vi "Main.vi"(9 "MICROS":T1, 10 "VISA resource name":refnum<visa-resource-name>, 11 "Module Admin":refnum<class "Delacor_lib_QMH_Cloneable Module Admin.lvclass">) -> ()   [LabVIEW 2019, in "MAIN.lvlib"]
doc: "This template is based off of the Queued Message Handler design pattern and the Queued Message Handler project template that ships with LabVIEW.\n\nThe main difference is that the queue is private to this module and communication between modules is performed via Broadcast and Request events.\n\nRequest events are wrapped in public API methods and are handled in the Event Handling Loop (EHL) of this VI. Any module can register for Broadcast events sent by this module. The EHL generates messages based on user interface actions.\n\nThe Message Handling Loop (MHL) processes messages generated by the EHL, or by other messages. The messages are string values, so new messages can be added easily to the Message Cases case structure in the MHL. Each message cluster can also provide an optional value for Message Data, which is a variant that can be converted to whatever message-specific data is required.\n_____\nBased on Delacor QMH Project Template 5.0.0.82."
uses:
  MAIN.lvlib
  <vilib>/Delacor/Delacor QMH/Libraries/Cloneable Module Admin_class/Delacor_lib_QMH_Cloneable Module Admin.lvclass
  C:/Program Files (x86)/National Instruments/LabVIEW 2019/vi.lib/Delacor/Delacor QMH/Libraries/Module Admin_class/Delacor_lib_QMH_Module Admin.lvclass
  MICROS.ctl
  Module Data--cluster.ctl
  ARDUINO/ARDUINO.lvclass
  D:/Repositorios Git/FINAL_AHORA_SI/SERIAL DEVICE/SERIAL DEVICE.lvclass
  <vilib>/Delacor/Delacor QMH/Libraries/Message Queue_class/Delacor_lib_QMH_Message Queue.lvclass/Delacor_lib_QMH_Message Queue.ctl
  <vilib>/Delacor/Delacor QMH/Libraries/Cloneable Module Admin_class/Delacor_lib_QMH_Cloneable Module Admin.lvclass/Delacor_lib_QMH_Cloneable Module Admin.ctl
  Stop Argument--cluster.ctl
  <vilib>/Delacor/Delacor QMH/Libraries/Module Admin_class/Delacor_lib_QMH_Module Admin.lvclass/Delacor_lib_QMH_Module Admin.ctl
  READ_ADC Argument--cluster.ctl
  READ_ADC (Reply Payload)--cluster.ctl
  READ PIN Argument--cluster.ctl
  READ PIN (Reply Payload)--cluster.ctl
  <vilib>/Utility/miscctls.llb/LVPointTypeDef.ctl
  SERIAL DEVICE/SERIAL DEVICE.lvclass/SERIAL DEVICE.ctl
  <vilib>/Delacor/Delacor QMH/Libraries/Message Queue_class/Delacor_lib_QMH_Enqueue Message (Single).vi
  <vilib>/Delacor/Delacor QMH/Libraries/Cloneable Module Admin_class/Delacor_lib_QMH_Get Module ID.vi
  <vilib>/Delacor/Delacor QMH/Libraries/Module Admin_class/Delacor_lib_QMH_Get External Launch.vi
  <vilib>/Utility/error.llb/Error Cluster From Error Code.vi
  <vilib>/ErrorRing/Error Ring.xnode
  <vilib>/Delacor/Delacor QMH/Libraries/Message Queue_class/Delacor_lib_QMH_Message Queue.lvclass
  SERIAL DEVICE/SERIAL DEVICE.lvclass
panel:
  out "Lectua PIN":string
  in  "Leer estado Pin":bool
  in  "Número de pin":u8
  in  "LEER ADC":bool
  out "LECTURA ADC":string
  in  "CANAL":u8
  in  "Simulate MHL Error":bool
  in  "Simulate EHL Error":bool
  out "error out":errorcluster
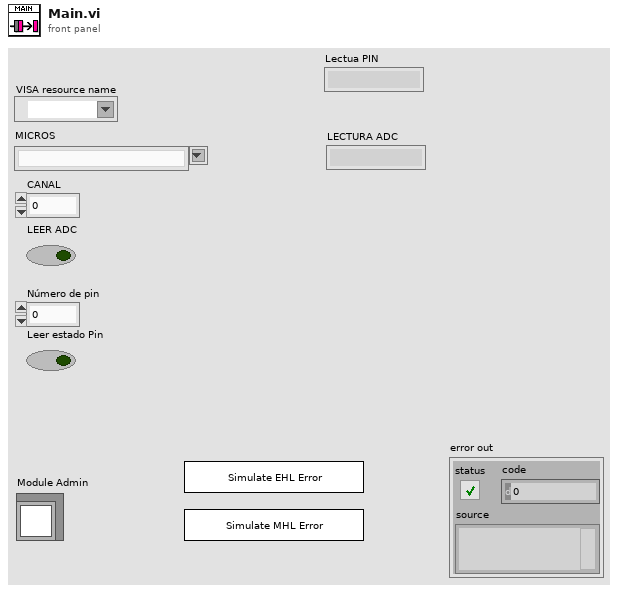
[diagram p1: front panel]
types:
  T1 = typedef "MICROS.ctl" = string
  T2 = typedef "MAIN.lvlib/Request Events--cluster.ctl" = cluster{"Stop Module":refnum<user-event>, "Show Panel":refnum<user-event>, "Hide Panel":refnum<user-event>, "Show Diagram":refnum<user-event>, "Get Module Execution Status":refnum<user-event>, "READ_ADC":refnum<user-event>, "READ PIN":refnum<user-event>}
  T3 = typedef "MAIN.lvlib/Module Data--cluster.ctl" = cluster{"Status":string, "SERIAL DEVICE":refnum<class "ARDUINO.lvclass">}
  T4 = enum32{"invalid lock state", "Not Locked", "Locked (No Password)", "Password-protected"}
  T5 = typedef "MAIN.lvlib/Stop Argument--cluster.ctl" = cluster{"Module ID":i32, "Origin":string, "Exit via Stop Module Req?":bool, "Wait for Module to stop?":bool}
  T6 = typedef "MAIN.lvlib/READ_ADC Argument--cluster.ctl" = cluster{"Module ID":i32, "CANAL":u8, "Wait Notifier":refnum<notifier>, "wait for reply":bool}
  T7 = typedef "MAIN.lvlib/READ PIN Argument--cluster.ctl" = cluster{"Module ID":i32, "CANAL PIN":u8, "Wait Notifier":refnum<notifier>, "wait for reply":bool}
  T8 = typedef "LVPointTypeDef.ctl" = cluster{"Horizontal":i16, "Vertical":i16}
  T9 = enum32{"Invalid", "Standard", "Closed", "Hidden", "Minimized", "Maximized"}
  T10 = typedef "MAIN.lvlib/READ_ADC (Reply Payload)--cluster.ctl" = cluster{"read buffer":string, "READ_ADC_error":errorcluster}
  T11 = typedef "MAIN.lvlib/READ PIN (Reply Payload)--cluster.ctl" = cluster{"READ BUFFER":string, "READ PIN_error":errorcluster}
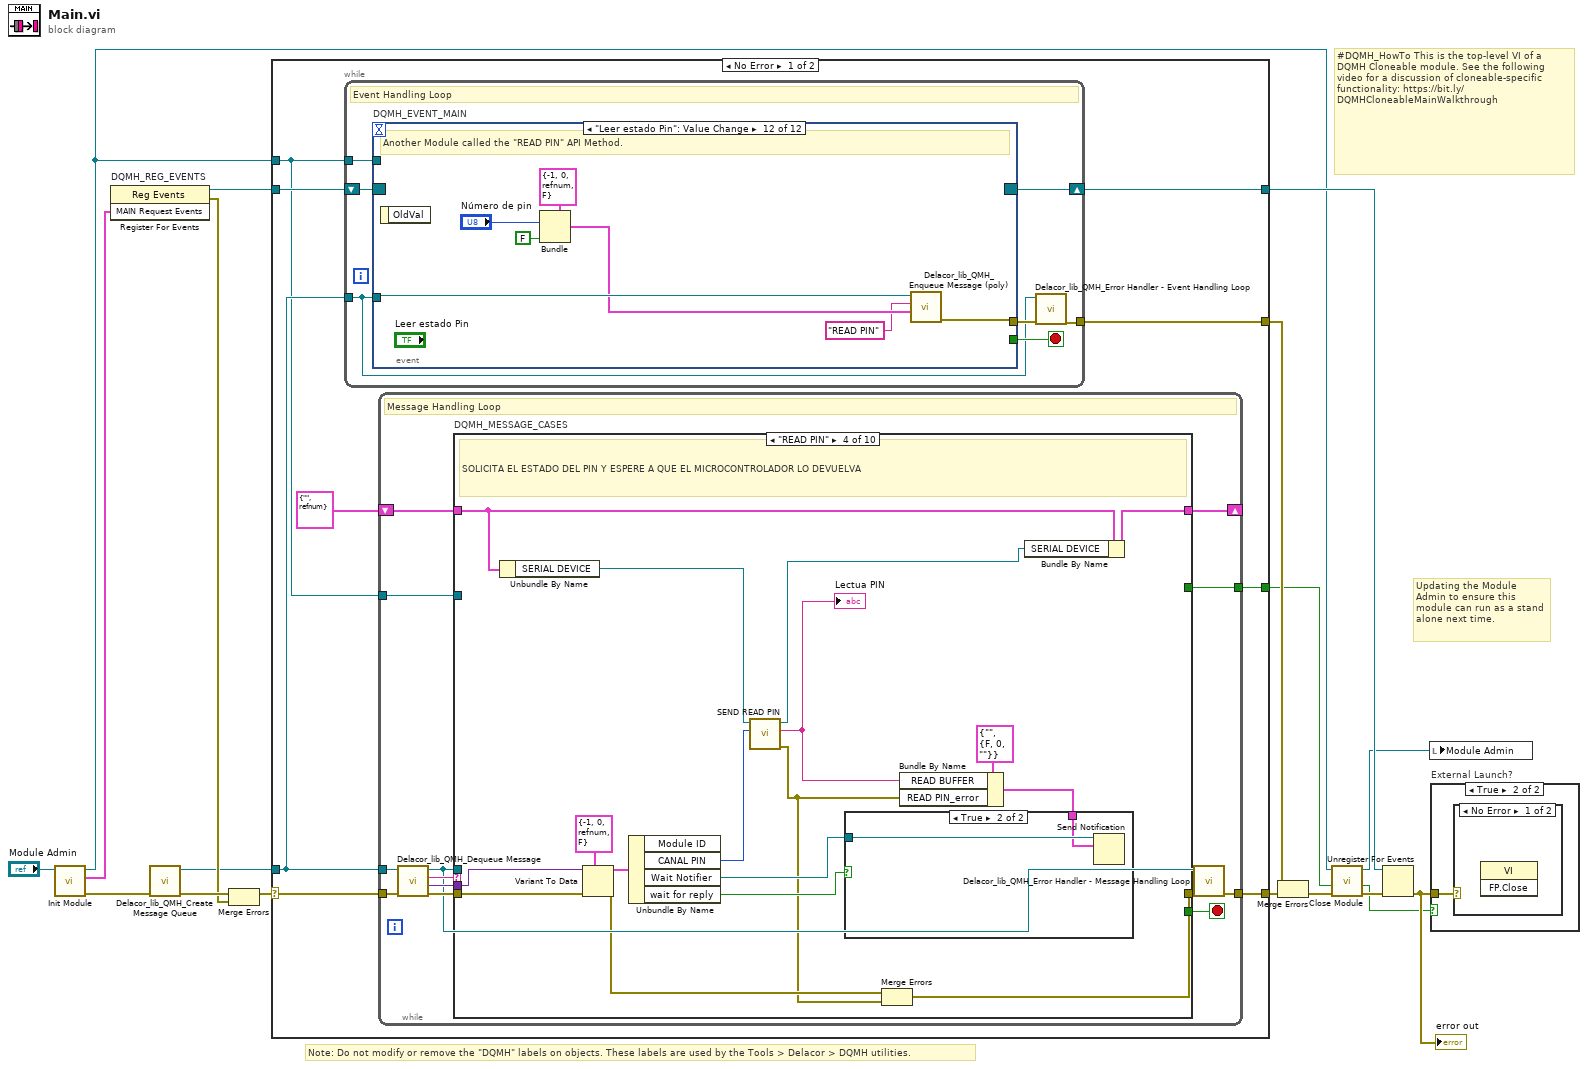
[diagram p0: block diagram]
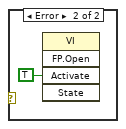
[diagram p3: hidden frame]
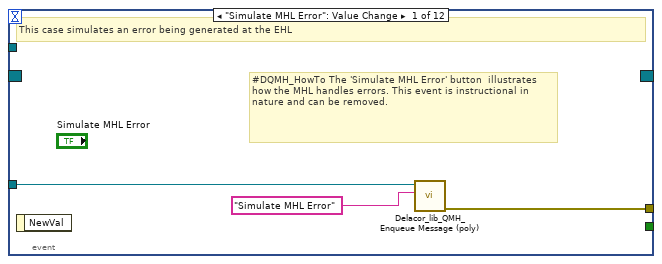
[diagram p4: hidden frame]
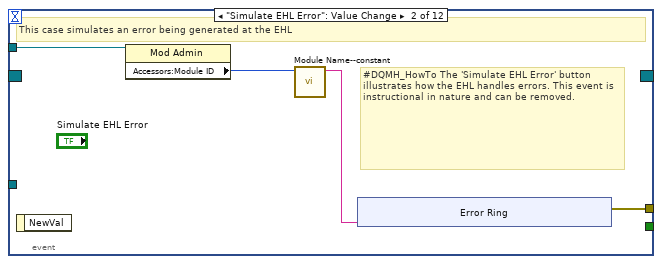
[diagram p5: hidden frame]
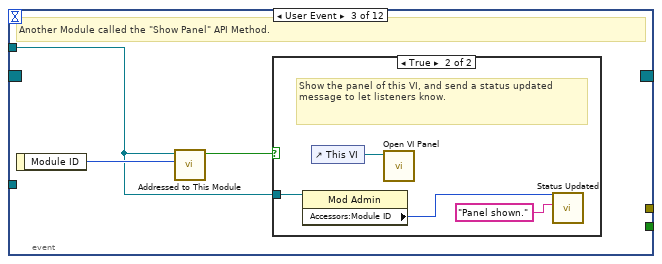
[diagram p6: hidden frame]
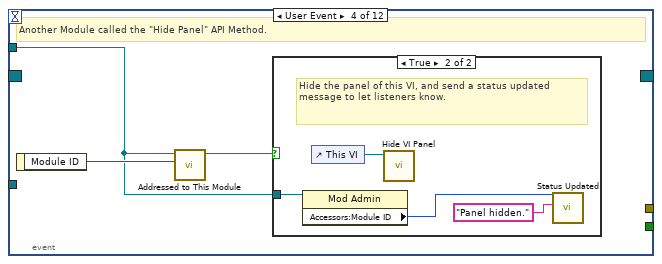
[diagram p8: hidden frame]
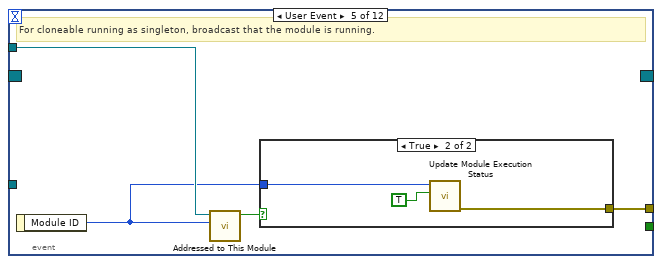
[diagram p10: hidden frame]
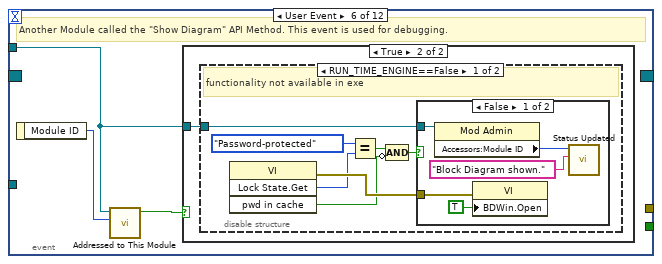
[diagram p12: hidden frame]
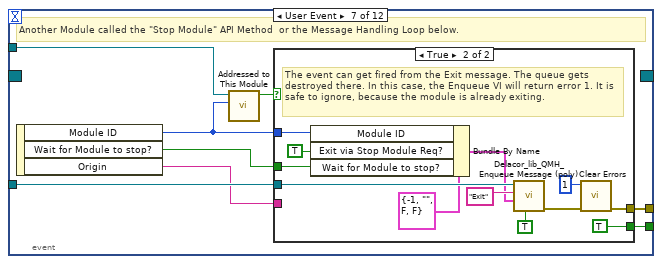
[diagram p16: hidden frame]
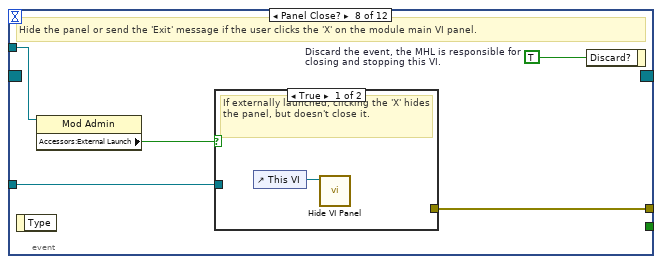
[diagram p18: hidden frame]
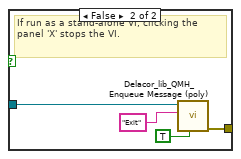
[diagram p19: hidden frame]
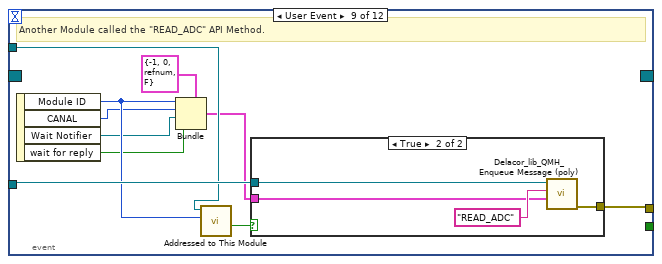
[diagram p20: hidden frame]
diagram:
  # "#DQMH_HowTo This is the top-level VI of a DQMH Cloneable module. See the following video for a discussion of cloneable-specific functionality: https://bit.ly/DQMHCloneableMainWalkthrough"
  # "Note: Do not modify or remove the \"DQMH\" labels on objects. These labels are used by the Tools > Delacor > DQMH utilities."
  # "Updating the Module Admin to ensure this module can run as a stand alone next time."
  n1 = call "Init Module.vi"("Cloneable Module Admin in"="Module Admin") -> ("error out"=w15:errorcluster, "MAIN Request Events"=w7:T2, "Cloneable Module Admin out"=w4:refnum<class "Delacor_lib_QMH_Cloneable Module Admin.lvclass">)  [unwired: 8 in]
  n2 = register-events "DQMH_REG_EVENTS"(w7) -> (reference out=w8:refnum<event-registration>, error out=w10:errorcluster)  [unwired: 2 in]
  n3 = call <vilib>:"Delacor_lib_QMH_Create Message Queue.vi"("error in (no error)"=w15) -> ("error out"=w12:errorcluster, "Message Queue"=w6:refnum<class "Delacor_lib_QMH_Message Queue.lvclass">)  [unwired: 9 in]
  n4 = Merge Errors(w12, w10) -> (w11:errorcluster)
  n5 = case shown="No Error" w11 {
    selector: w11 -> [w25 w313]
    tunnel: [w27 w312] -> w16
    tunnel: [w24 w320] -> w9
    tunnel: w8 -> [w22 w320]
    tunnel: w6 -> [w21 w311]
    tunnel: [w26 _] -> w17
    tunnel: w4 -> [w20 w316]
    tunnel: [w19 _] -> w2
    frame No Error {
      n6 = while {
        tunnel: w21 -> [w28]
        shift-right: [w31] -> w24
        shift-left: w22 -> [w32]
        tunnel: [w33] -> w26
        tunnel: w20 -> [w29]
        stop <- w30 stop-if-true
        # "Event Handling Loop"
        n7 = event "DQMH_EVENT_MAIN" shown="[11] \"Leer estado Pin\": Value Change" {
          selector: w32 -> [_ _ _ _ _ _ _ _ _ _ _ _]
          dyn-events: [_ _ _ _ _ _ _ _ _ _ _ _] -> w31
          timeout: _ -> [_ _ _ _ _ _ _ _ _ _ _ _]
          tunnel: [_ _ _ _ _ _ w89 _ _ _ _ _] -> w30
          tunnel: w28 -> [w36 _ _ _ _ _ w92 w107 w125 w136 w146 w157]
          tunnel: [w37 w41 _ _ w66 _ w93 w110 w116 w133 w137 w154] -> w34
          tunnel: w29 -> [_ w40 w49 w56 w64 w70 w91 w108 w123 _ w144 _]
          event "Simulate MHL Error": Value Change {
            # "#DQMH_HowTo The 'Simulate MHL Error' button  illustrates how the MHL handles errors. This event is instructional in nature and can be removed."
            # "This case simulates an error being generated at the EHL"
            n8 = event-data() -> ()  [unwired: 1 in, 1 out]
            n9 = call-poly <vilib>:"Delacor_lib_QMH_Enqueue Message (poly).vi"("Message"="Simulate MHL Error", "Message Queue in"=w36) -> ("error out"=w37:errorcluster)  [unwired: 8 in, 1 out]
          }
          event "Simulate EHL Error": Value Change {
            # "#DQMH_HowTo The 'Simulate EHL Error' button  illustrates how the EHL handles errors. This event is instructional in nature and can be removed."
            # "This case simulates an error being generated at the EHL"
            n10 = event-data() -> ()  [unwired: 1 in, 1 out]
            n11 = property class="Mod Admin"(reference=w40) -> ("Accessors:Module ID"=w39:i32)  [unwired: 1 in, 2 out]
            n12 = call "Module Name--constant.vi"("Module ID"=w39) -> ("Module Name"=w38:string)  [unwired: 10 in]
            n13 = xnode "Error Ring"("parameter 0"=w38) -> ("error out"=w41:errorcluster)
          }
          event User Event {
            # "Another Module called the \"Show Panel\" API Method."
            n14 = event-data() -> ("Module ID"=w50:i32)  [unwired: 1 in]
            n15 = call "Addressed to This Module.vi"("Module ID from Argument"=w50, "Module Admin"=w49) -> ("Addressed to this instance?"=w51:bool)  [unwired: 8 in, 1 out]
            n16 = case shown="True" w51 {
              tunnel: w49 -> [_ w53]
              frame False {
              }
              frame True {
                # "Show the panel of this VI, and send a status updated message to let listeners know."
                n17 = property class="Mod Admin"(reference=w53) -> ("Accessors:Module ID"=w52:i32)  [unwired: 1 in, 2 out]
                n18 = control-ref of="This VI"() -> (w55:refnum<vi>)
                n19 = call "Open VI Panel.vi"("VI"=w55) -> ()  [unwired: 10 in, 1 out]
                n20 = call "Status Updated.vi"("Status"="Panel shown." ("format string"), "Module ID"=w52) -> ()  [unwired: 9 in, 1 out]
              }
            }
          }
          event User Event {
            # "Another Module called the \"Hide Panel\" API Method."
            n21 = event-data() -> ("Module ID"=w57:i32)  [unwired: 1 in]
            n22 = call "Addressed to This Module.vi"("Module ID from Argument"=w57, "Module Admin"=w56) -> ("Addressed to this instance?"=w58:bool)  [unwired: 8 in, 1 out]
            n23 = case shown="True" w58 {
              tunnel: w56 -> [_ w60]
              frame False {
              }
              frame True {
                # "Hide the panel of this VI, and send a status updated message to let listeners know."
                n24 = property class="Mod Admin"(reference=w60) -> ("Accessors:Module ID"=w59:i32)  [unwired: 1 in, 2 out]
                n25 = control-ref of="This VI"() -> (w62:refnum<vi>)
                n26 = call "Hide VI Panel.vi"("VI"=w62) -> ()  [unwired: 10 in, 1 out]
                n27 = call "Status Updated.vi"("Status"="Panel hidden." ("format string"), "Module ID"=w59) -> ()  [unwired: 9 in, 1 out]
              }
            }
          }
          event User Event {
            # "For cloneable running as singleton, broadcast that the module is running."
            n28 = event-data() -> ("Module ID"=w63:i32)  [unwired: 1 in]
            n29 = call "Addressed to This Module.vi"("Module ID from Argument"=w63, "Module Admin"=w64) -> ("Addressed to this instance?"=w65:bool)  [unwired: 8 in, 1 out]
            n30 = case shown="True" w65 {
              tunnel: [_ w69] -> w66
              tunnel: w63 -> [_ w68]
              frame False {
              }
              frame True {
                n31 = call "Update Module Execution Status.vi"("Running?"=TRUE, "Module ID"=w68) -> ("error out"=w69:errorcluster)  [unwired: 9 in]
              }
            }
          }
          event User Event {
            # "Another Module called the \"Show Diagram\" API Method. This event is used for debugging."
            n32 = event-data() -> ("Module ID"=w71:i32)  [unwired: 1 in]
            n33 = call "Addressed to This Module.vi"("Module ID from Argument"=w71, "Module Admin"=w70) -> ("Addressed to this instance?"=w72:bool)  [unwired: 8 in, 1 out]
            n34 = case shown="True" w72 {
              tunnel: w70 -> [_ w73]
              frame False {
              }
              frame True {
                n35 = disable-structure shown="RUN_TIME_ENGINE==False" {
                  disable-tunnel: w73 -> [w74 _]
                  frame condition #0 (active) {
                    # "functionality not available in exe"
                    n36 = invoke class="VI" method="Lock State.Get"() -> (error out=w80:errorcluster, "Get Lock State"=w79:T4, "pwd in cache"=w76:bool)  [unwired: 4 in, 1 out]
                    n37 = Equal?(x=T4."Password-protected", y=w79) -> (x = y?=w77:bool)
                    n38 = Compound Arithmetic op=AND(w77, invert w76) -> (w75:bool)
                    n39 = case shown="False" w75 {
                      tunnel: w80 -> [w85 _]
                      tunnel: w74 -> [w82 _]
                      frame False {
                        n40 = property class="Mod Admin"(reference=w82) -> ("Accessors:Module ID"=w81:i32)  [unwired: 1 in, 2 out]
                        n41 = property class="VI"(error in=w85, "BDWin.Open"=TRUE ("Block Diagram Window:Open")) -> ()  [unwired: 1 in, 2 out]
                        n42 = call "Status Updated.vi"("Status"="Block Diagram shown." ("format string"), "Module ID"=w81) -> ()  [unwired: 9 in, 1 out]
                      }
                      frame True {
                        # "Password-protected VI, and the password is not in the cache. Do not show the diagram."
                      }
                    }
                  }
                  frame condition #1 {
                  }
                }
              }
            }
          }
          event User Event {
            # "Another Module called the \"Stop Module\" API Method  or the Message Handling Loop below."
            n43 = event-data() -> ("Module ID"=w87:i32, "Wait for Module to stop?"=w88:bool, "Origin"=w86:string)  [unwired: 1 in]
            n44 = call "Addressed to This Module.vi"("Module ID from Argument"=w87, "Module Admin"=w91) -> ("Addressed to this instance?"=w90:bool)  [unwired: 8 in, 1 out]
            n45 = case shown="True" w90 {
              tunnel: [_ w104] -> w93
              tunnel: w92 -> [_ w100]
              tunnel: [_ TRUE] -> w89
              tunnel: w88 -> [_ w95]
              tunnel: w87 -> [_ w97]
              tunnel: w86 -> [_ _]
              frame False {
              }
              frame True {
                # "The event can get fired from the Exit message. The queue gets destroyed there. In this case, the Enqueue VI will return error 1. It is safe to ignore, because the module is already exiting."
                n46 = Bundle By Name(cluster=T5 {"Module ID"=-1, "Origin"="", "Exit via Stop Module Req?"=FALSE, "Wait for Module to stop?"=FALSE} ("Stop Argument"), "Module ID"=w97, "Exit via Stop Module Req?"=TRUE, "Wait for Module to stop?"=w95) -> (w94:T5)
                n47 = call-poly <vilib>:"Delacor_lib_QMH_Enqueue Message (poly).vi"("Priority Message? (F)"=TRUE, "Message Data"=w94, "Message"="Exit", "Message Queue in"=w100) -> ("error out"=w105:errorcluster)  [unwired: 6 in, 1 out]
                n48 = call <vilib>:"Clear Errors.vi"("error in (no error)"=w105, "specific error code to clear (0: all)"=1) -> ("error out"=w104:errorcluster)  [unwired: 4 in, 1 out]
              }
            }
          }
          event Panel Close? {
            w109 = TRUE  # Discard the event, the MHL is responsible for closing and stopping this VI.
            # "Hide the panel or send the 'Exit' message if the user clicks the 'X' on the module main VI panel."
            n49 = event-data() -> ()  [unwired: 1 in, 1 out]
            n50 = property class="Mod Admin"(reference=w108) -> ("Accessors:External Launch"=w106:bool)  [unwired: 1 in, 2 out]
            n51 = case shown="True" w106 {
              tunnel: w107 -> [_ w114]
              tunnel: [_ w115] -> w110
              frame True {
                # "If externally launched, clicking the 'X' hides the panel, but doesn't close it."
                n52 = control-ref of="This VI"() -> (w111:refnum<vi>)
                n53 = call "Hide VI Panel.vi"("VI"=w111) -> ()  [unwired: 10 in, 1 out]
              }
              frame False {
                # "If run as a stand-alone VI, clicking the panel 'X' stops the VI."
                n54 = call-poly <vilib>:"Delacor_lib_QMH_Enqueue Message (poly).vi"("Priority Message? (F)"=TRUE, "Message"="Exit", "Message Queue in"=w114) -> ("error out"=w115:errorcluster)  [unwired: 7 in, 1 out]
              }
            }
            n55 = event-data("Discard?"=w109) -> ()  [unwired: 1 in, 1 out]
          }
          event User Event {
            # "Another Module called the \"READ_ADC\" API Method."
            n56 = event-data() -> ("Module ID"=w120:i32, "CANAL"=w119:u8, "Wait Notifier"=w118:refnum<notifier>, "wait for reply"=w117:bool)  [unwired: 1 in]
            n57 = Bundle(cluster=T6 {"Module ID"=-1, "CANAL"=0, "Wait Notifier"=refnum, "wait for reply"=FALSE} ("READ_ADC Argument"), "Module ID"=w120, "CANAL"=w119, "Wait Notifier"=w118, "wait for reply"=w117) -> (w121:T6)
            n58 = call "Addressed to This Module.vi"("Module ID from Argument"=w120, "Module Admin"=w123) -> ("Addressed to this instance?"=w124:bool)  [unwired: 8 in, 1 out]
            n59 = case shown="True" w124 {
              tunnel: w125 -> [_ w129]
              tunnel: w121 -> [_ w127]
              tunnel: [_ w126] -> w116
              frame False {
              }
              frame True {
                n60 = call-poly <vilib>:"Delacor_lib_QMH_Enqueue Message (poly).vi"("Message Data"=w127, "Message"="READ_ADC", "Message Queue in"=w129) -> ("error out"=w126:errorcluster)  [unwired: 7 in, 1 out]
              }
            }
          }
          event "LEER ADC": Value Change {
            # "Another Module called the \"READ_ADC\" API Method."
            n61 = event-data() -> ()  [unwired: 1 in, 2 out]
            n62 = Bundle(cluster=T6 {"Module ID"=-1, "CANAL"=0, "Wait Notifier"=refnum, "wait for reply"=FALSE} ("READ_ADC Argument"), "CANAL"="CANAL", "wait for reply"=FALSE) -> (w134:T6)  [unwired: 2 in]
            n63 = call-poly <vilib>:"Delacor_lib_QMH_Enqueue Message (poly).vi"("Message Data"=w134, "Message"="READ_ADC", "Message Queue in"=w136) -> ("error out"=w133:errorcluster)  [unwired: 7 in, 1 out]
          }
          event User Event {
            # "Another Module called the \"READ PIN\" API Method."
            n64 = event-data() -> ("Module ID"=w141:i32, "CANAL PIN"=w140:u8, "Wait Notifier"=w139:refnum<notifier>, "wait for reply"=w138:bool)  [unwired: 1 in]
            n65 = Bundle(cluster=T7 {"Module ID"=-1, "CANAL PIN"=0, "Wait Notifier"=refnum, "wait for reply"=FALSE} ("READ PIN Argument"), "Module ID"=w141, "CANAL PIN"=w140, "Wait Notifier"=w139, "wait for reply"=w138) -> (w142:T7)
            n66 = call "Addressed to This Module.vi"("Module ID from Argument"=w141, "Module Admin"=w144) -> ("Addressed to this instance?"=w145:bool)  [unwired: 8 in, 1 out]
            n67 = case shown="True" w145 {
              tunnel: w146 -> [_ w150]
              tunnel: w142 -> [_ w148]
              tunnel: [_ w147] -> w137
              frame False {
              }
              frame True {
                n68 = call-poly <vilib>:"Delacor_lib_QMH_Enqueue Message (poly).vi"("Message Data"=w148, "Message"="READ PIN", "Message Queue in"=w150) -> ("error out"=w147:errorcluster)  [unwired: 7 in, 1 out]
              }
            }
          }
          event "Leer estado Pin": Value Change {
            # "Another Module called the \"READ PIN\" API Method."
            n69 = event-data() -> ()  [unwired: 1 in, 1 out]
            n70 = Bundle(cluster=T7 {"Module ID"=-1, "CANAL PIN"=0, "Wait Notifier"=refnum, "wait for reply"=FALSE} ("READ PIN Argument"), "CANAL PIN"="Número de pin", "wait for reply"=FALSE) -> (w155:T7)  [unwired: 2 in]
            n71 = call-poly <vilib>:"Delacor_lib_QMH_Enqueue Message (poly).vi"("Message Data"=w155, "Message"="READ PIN", "Message Queue in"=w157) -> ("error out"=w154:errorcluster)  [unwired: 7 in, 1 out]
          }
        }
        n72 = call-dynamic "Delacor_lib_QMH_Error Handler - Event Handling Loop.vi"("error in (no error)"=w34, "Message Queue in"=w28) -> ("dup error in"=w33:errorcluster)  [unwired: 8 in, 1 out]
      }
      n73 = while {
        tunnel: w21 -> [w161]
        shift-right: [w165] -> _
        shift-left: T3 {"Status"="", "SERIAL DEVICE"=refnum} ("Data Cluster") -> [w166]
        tunnel: w25 -> [w169]
        tunnel: [w167] -> w27
        tunnel: w20 -> [w159]
        tunnel: [w158] -> w19
        stop <- w164 stop-if-true
        # "Message Handling Loop"
        n74 = call-dynamic "Delacor_lib_QMH_Dequeue Message.vi"("error in (no error)"=w169, "Message Queue in"=w161) -> ("error out"=w168:errorcluster, "Message Data"=w162:variant, "Message"=w163:string, "Message Queue out"=w160:refnum<class "Delacor_lib_QMH_Message Queue.lvclass">)  [unwired: 6 in]
        n75 = case "DQMH_MESSAGE_CASES" shown="\"READ PIN\"" w163 {
          selector: w163 -> [_ _ _ _ _ _ _ _ _ w298]
          tunnel: w160 -> [_ _ _ _ _ _ w248 _ w288 _]
          tunnel: w168 -> [w195 w200 w219 w238 w243 w245 w257 w270 w294 w300]
          tunnel: [w193 w200 w210 w229 w242 w245 w253 w269 w291 w301] -> w170
          tunnel: w166 -> [w186 w199 w206 w227 w241 w244 w252 w267 w279 w299]
          tunnel: [w185 w199 w205 w228 w241 w244 w252 w267 w279 w299] -> w165
          tunnel: [_ _ _ _ _ _ _ _ w287 _] -> w164
          tunnel: w162 -> [_ _ w217 w236 _ _ w251 _ w285 _]
          tunnel: w159 -> [w180 _ _ _ _ _ w250 w265 w281 w296]
          tunnel: [_ _ _ _ _ _ _ _ w283 _] -> w158
          frame "Initialize" {
            # "Initialize - Any operation that needs to be done before the module can receive messages. Synchronize Caller Events.vi will inform Start Module.vi that the module has launched and is ready to receive messages. Module Did Init.vi will broadcast that the module initialized."
            n76 = call "Synchronize Caller Events.vi"("error in (no error)"=w195, "Module Admin"=w180) -> ("error out"=w194:errorcluster, "Module Admin out"=w179:refnum<class "Delacor_lib_QMH_Cloneable Module Admin.lvclass">)  [unwired: 8 in]
            n77 = property class="Mod Admin"(reference=w179) -> ("Accessors:Module ID"=w182:i32, "Accessors:External Launch"=w181:bool)  [unwired: 1 in, 2 out]
            n78 = case shown="\"A\"" "MICROS" {
              tunnel: [_ refnum<class "ARDUINO.lvclass"> refnum ("ARDUINO.lvclass")] -> w177
              frame "False", Default {
              }
              frame "A" {
              }
            }
            n79 = call "Module Name--constant.vi"("Module ID"=w182) -> ("Module Name"=w190:string)  [unwired: 10 in]
            n80 = call "Write MICROS.vi"("MICROS"="MICROS", "SERIAL DEVICE in"=w177) -> ("SERIAL DEVICE out"=w175:refnum<class "ARDUINO.lvclass">)  [unwired: 8 in, 1 out]
            n81 = property class="VI"("Front Panel.Title"=w190) -> (reference out=w192:refnum<vi>, error out=w197:errorcluster)  [unwired: 2 in]
            n82 = Select(t=T9."Hidden" ("State"), s=w181, f=T9."Standard" ("State")) -> (s? t:f=w187:T9)
            n83 = VISA Open(VISA resource name="VISA resource name") -> (VISA resource name=w171:refnum<visa-resource-name>)  [unwired: 4 in, 1 out]
            n84 = invoke class="VI" method="FP.Open"(reference=w192, error in=w197, "State"=w187) -> (reference out=w191:refnum<vi>, error out=w196:errorcluster)  [unwired: 2 in, 3 out]
            n85 = call "Module Name--constant.vi"("Module ID"=w182) -> ("Module Name"=w183:string)  [unwired: 10 in]
            n86 = call "Write VISA resource name.vi"("VISA resource name"=w171, "SERIAL DEVICE in"=w175) -> ("SERIAL DEVICE out"=w174:refnum<class "ARDUINO.lvclass">)  [unwired: 8 in, 1 out]
            n87 = call-dynamic "INIT.vi"("SERIAL DEVICE in"=w174) -> ("SERIAL DEVICE out"=w172:refnum<class "ARDUINO.lvclass">)  [unwired: 9 in, 1 out]
            n88 = invoke class="VI" method="FP.Center"(reference=w191, error in=w196) -> ()  [unwired: 1 in, 3 out]
            n89 = call "Module Did Init.vi"("error in (no error)"=w194, "Initialized?"=TRUE, "Origin"=w183, "Module ID"=w182) -> ("error out"=w193:errorcluster)  [unwired: 7 in]
            n90 = Bundle By Name(cluster=w186, "SERIAL DEVICE"=w172) -> (w185:T3)
            n91 = property on="Pane" class="Pane"("Origin"=T8 {"Horizontal"=0, "Vertical"=0}) -> ()  [unwired: 2 in, 2 out]
          }
          frame "--- Module Specific ---" {
            # "Separator -- The following cases handle messages specific to this Module."
          }
          frame "READ_ADC" {
            # "MANDA LEER EL ADC Y ESPERA A QUE EL MICRO RESPONDA LO ESPERADO"
            n92 = Unbundle By Name(w206) -> ("SERIAL DEVICE"=w207:refnum<class "ARDUINO.lvclass">)
            n93 = Variant To Data(error in=w219, type=T6 {"Module ID"=-1, "CANAL"=0, "Wait Notifier"=refnum, "wait for reply"=FALSE} ("READ_ADC Argument"), Variant=w217) -> (data=w215:T6, error out=w218:errorcluster)
            n94 = Unbundle By Name(w215) -> ("CANAL"=w209:u8, "Wait Notifier"=w214:refnum<notifier>, "wait for reply"=w213:bool)  [unwired: 1 out]
            n95 = call-dynamic "SEND ADC.vi"("CANAL"=w209, "SERIAL DEVICE in"=w207) -> ("error out"=w208:errorcluster, "read buffer"=w203:string, "SERIAL DEVICE out"=w204:refnum<class "ARDUINO.lvclass">)  [unwired: 7 in]
            n96 = Match Pattern(string=w203, regular expression=";") -> (before substring=→"LECTURA ADC":string)  [unwired: 1 in, 3 out]
            n97 = Bundle By Name(cluster=T10 {"read buffer"="", "READ_ADC_error"={"status"=FALSE, "code"=0, "source"=""}} ("READ_ADC (Reply Payload)"), "read buffer"=w203, "READ_ADC_error"=w208) -> (w212:T10)
            n98 = case shown="True" w213 {
              tunnel: w214 -> [_ w221]
              tunnel: w212 -> [_ w220]
              frame False {
              }
              frame True {
                n99 = Send Notification(notification=w220, notifier=w221) -> ()  [unwired: 1 in, 2 out]
              }
            }
            n100 = Merge Errors(w218, w208) -> (w210:errorcluster)
            n101 = Bundle By Name(cluster=w206, "SERIAL DEVICE"=w204) -> (w205:T3)
          }
          frame "READ PIN" {
            # "SOLICITA EL ESTADO DEL PIN Y ESPERE A QUE EL MICROCONTROLADOR LO DEVUELVA"
            n102 = Unbundle By Name(w227) -> ("SERIAL DEVICE"=w224:refnum<class "ARDUINO.lvclass">)
            n103 = Variant To Data(error in=w238, type=T7 {"Module ID"=-1, "CANAL PIN"=0, "Wait Notifier"=refnum, "wait for reply"=FALSE} ("READ PIN Argument"), Variant=w236) -> (data=w234:T7, error out=w237:errorcluster)
            n104 = Unbundle By Name(w234) -> ("CANAL PIN"=w223:u8, "Wait Notifier"=w233:refnum<notifier>, "wait for reply"=w232:bool)  [unwired: 1 out]
            n105 = call-dynamic "SEND READ PIN.vi"("CANAL"=w223, "SERIAL DEVICE in"=w224) -> ("error out"=w222:errorcluster, "read buffer"=w226:string, "SERIAL DEVICE out"=w225:refnum<class "ARDUINO.lvclass">)  [unwired: 7 in]
            "Lectua PIN" <- w226
            n106 = Merge Errors(w237, w222) -> (w229:errorcluster)
            n107 = Bundle By Name(cluster=T11 {"READ BUFFER"="", "READ PIN_error"={"status"=FALSE, "code"=0, "source"=""}} ("READ PIN (Reply Payload)"), "READ BUFFER"=w226, "READ PIN_error"=w222) -> (w231:T11)
            n108 = case shown="True" w232 {
              tunnel: w233 -> [_ w240]
              tunnel: w231 -> [_ w239]
              frame False {
              }
              frame True {
                n109 = Send Notification(notification=w239, notifier=w240) -> ()  [unwired: 1 in, 2 out]
              }
            }
            n110 = Bundle By Name(cluster=w227, "SERIAL DEVICE"=w225) -> (w228:T3)
          }
          frame "---Copy This Frame---" {
            # "Duplicate this frame when creating new messages.  Change this comment in the duplicated frame to describe this message."
            n111 = Merge Errors(w243) -> (w242:errorcluster)
          }
          frame "--- Exit and Error Handling---" {
            # "Separator - the following cases handle errors and exit messages."
          }
          frame "Error" {
            # "#CodeRecommended - If you ever change the name of this \"Error\" message, you'll need to update the name in the Check Loop Error.vi as well."
            # "#CodeRecommended - If the module is running in standalone mode (External Launch = FALSE), this code will pop up an error dialog and call the 'Exit' message if an error occurs. Add more fine-grained error handling here."
            # "Error - Check the error message data and respond accordingly. This message is sent by the \"Error Handler\" VIs at the end of each loop in this application."
            n112 = property class="Mod Admin"(reference=w250) -> ("Accessors:External Launch"=w249:bool, "Accessors:Module ID"=w246:i32)  [unwired: 1 in, 2 out]
            n113 = Variant To Data(error in=w257, type=errorcluster {"status"=FALSE, "code"=0, "source"=""} ("error constant"), Variant=w251) -> (data=w258:errorcluster, error out=w255:errorcluster)
            n114 = call "Module Name--constant.vi"("Module ID"=w246) -> ("Module Name"=w247:string)  [unwired: 10 in]
            n115 = call "Error Reported.vi"("Additional Information"=w247, "Error"=w258, "Module ID"=w246) -> ()  [unwired: 8 in, 1 out]
            n116 = case shown="False" w249 {
              tunnel: [w263 _] -> w254
              tunnel: w248 -> [w261 _]
              tunnel: w258 -> [w262 _]
              frame False {
                # "If the module is running standalone, then pop up an error dialog and call the \"Exit\" message."
                n117 = call <vilib>:"Simple Error Handler.vi"("error in (no error)"=w262) -> ()  [unwired: 4 in, 5 out]
                n118 = call-poly <vilib>:"Delacor_lib_QMH_Enqueue Message (poly).vi"("Priority Message? (F)"=TRUE, "Message"="Exit", "Message Queue in"=w261) -> ("error out"=w263:errorcluster)  [unwired: 7 in, 1 out]
              }
              frame True {
                # "If the module was launched externally, calling the Error Reported broadcast VI is the only action performed by the \"Error\" message. The module's caller can then process the error appropriately."
              }
            }
            n119 = Merge Errors(w255, w254) -> (w253:errorcluster)
            n120 = local write "error out"(w253) -> ()
          }
          frame "Simulate MHL Error" {
            # "#DQMH_HowTo The 'Simulate MHL Error' button  illustrates how the MHL handles errors. This event is instructional in nature and can be removed."
            # "Simulate an error occurring at the MHL"
            n121 = property class="Mod Admin"(reference=w265) -> ("Accessors:Module ID"=w266:i32)  [unwired: 1 in, 2 out]
            n122 = call "Module Name--constant.vi"("Module ID"=w266) -> ("Module Name"=w264:string)  [unwired: 10 in]
            n123 = xnode "Error Ring"("parameter 0"=w264) -> ("error out"=w268:errorcluster)
            n124 = Merge Errors(w270, w268) -> (w269:errorcluster)
          }
          frame "Exit" {
            w286 = 91  # 91: not all Exit messages will have an argument
            w287 = TRUE  # Stop the VI
            # "Release the message queue reference"
            # "Exit - Exit the application."
            n125 = Variant To Data(error in=w294, type=T5 {"Module ID"=-1, "Origin"="", "Exit via Stop Module Req?"=FALSE, "Wait for Module to stop?"=FALSE} ("Stop Argument"), Variant=w285) -> (data=w282:T5, error out=w289:errorcluster)
            n126 = Unbundle By Name(w279) -> ("SERIAL DEVICE"=w278:refnum<class "ARDUINO.lvclass">)
            n127 = call <vilib>:"Clear Errors.vi"("error in (no error)"=w289, "specific error code to clear (0: all)"=w286) -> ("error out"=w293:errorcluster)  [unwired: 4 in, 1 out]
            n128 = call-dynamic "CLOSE.vi"("SERIAL DEVICE in"=w278) -> ()  [unwired: 9 in, 2 out]
            n129 = control-ref of="This VI"() -> (w280:refnum<vi>)
            n130 = call-dynamic "Delacor_lib_QMH_Release Message Queue.vi"("error in (no error)"=w293, "Message Queue"=w288) -> ("error out"=w292:errorcluster)  [unwired: 9 in]
            n131 = call "Handle Exit.vi"("Stop Argument"=w282, "Module Admin in"=w281, "VI reference"=w280) -> ("error out"=w290:errorcluster, "Wait for Stop?"=w283:bool)  [unwired: 7 in]
            n132 = Merge Errors(w292, w290) -> (w291:errorcluster)
          }
          frame Default {
            # "'Default' case only runs if there is a message that isn't defined in any of the other cases.  Output a programming error."
            n133 = property class="Mod Admin"(reference=w296) -> ("Accessors:Module ID"=w295:i32)  [unwired: 1 in, 2 out]
            n134 = call "Module Name--constant.vi"("Module ID"=w295) -> ("Module Name"=w297:string)  [unwired: 10 in]
            n135 = xnode "Error Ring"("parameter 0"=w298, "parameter 1"=w297) -> ("error out"=w302:errorcluster)
            n136 = Merge Errors(w300, w302) -> (w301:errorcluster)
          }
        }
        n137 = call-dynamic "Delacor_lib_QMH_Error Handler - Message Handling Loop.vi"("error in (no error)"=w170, "Message Queue in"=w160) -> ("dup error in"=w167:errorcluster)  [unwired: 8 in, 1 out]
      }
    }
    frame Error {
      n138 = call "Synchronize Caller Events.vi"("Module Admin"=w316) -> ("Module Admin out"=w315:refnum<class "Delacor_lib_QMH_Cloneable Module Admin.lvclass">)  [unwired: 9 in, 1 out]
      n139 = property class="Mod Admin"(reference=w315) -> ("Accessors:Module ID"=w314:i32)  [unwired: 1 in, 2 out]
      n140 = call-dynamic "Delacor_lib_QMH_Release Message Queue.vi"("error in (no error)"=w313, "Message Queue"=w311) -> ("error out"=w312:errorcluster)  [unwired: 9 in]
      n141 = call "Module Name--constant.vi"("Module ID"=w314) -> ("Module Name"=w319:string)  [unwired: 10 in]
      n142 = Format Into String(format string="An error occurred during initialization. %s is no longer running.", w319) -> (resulting string=w317:string)  [unwired: 2 in, 1 out]
      n143 = call "Error Reported.vi"("Additional Information"=w317, "Error"=w312, "Module ID"=w314) -> ()  [unwired: 8 in, 1 out]
    }
  }
  n144 = Merge Errors(w17, w16) -> (w18:errorcluster)
  n145 = call "Close Module.vi"("error in"=w18, "Wait for stop?"=w2, "Module Admin in"=w4) -> ("error out"=w14:errorcluster, "External Launch"=w1:bool, "Module Admin out"=w3:refnum<class "Delacor_lib_QMH_Cloneable Module Admin.lvclass">)  [unwired: 6 in]
  n146 = Unregister For Events(event registration refnum=w9, error in=w14) -> (error out=w13:errorcluster)
  "error out" <- w13
  n147 = local write "Module Admin"(w3) -> ()
  n148 = case "External Launch?" shown="True" w1 {
    tunnel: w13 -> [_ w321]
    frame False {
    }
    frame True {
      n149 = case shown="No Error" w321 {
        frame No Error {
          n150 = invoke class="VI" method="FP.Close"() -> ()  [unwired: 3 in, 3 out]
        }
        frame Error {
          n151 = invoke class="VI" method="FP.Open"("Activate"=TRUE ("Activate?")) -> ()  [unwired: 4 in, 5 out]
        }
      }
    }
  }
